vi "CheckKinect.vi"(8 "error in":errorcluster) -> (0 "error out":errorcluster, 2 "Hot?":bool)   [LabVIEW 2013]
doc: "Uses the Kinect to signal to the robot whether the goal is hot or not. If hands are detected, the goal is hot. Otherwise, the goal is not hot."
uses:
  <vilib>/addons/Kinect/Skeleton Vertex Index.ctl
  <vilib>/addons/Kinect/SkeletonVertexTrackState.ctl
panel:
  out "HandRightZ":sgl
  out "HandLeftZ":sgl
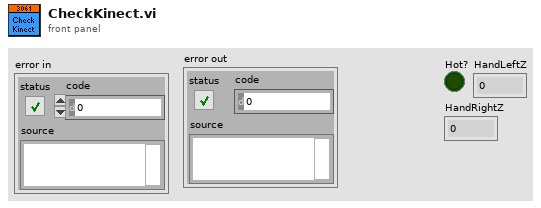
[diagram p1: front panel]
types:
  T1 = typedef "SkeletonVertexTrackState.ctl" = enum32{"NotTracked", "Inferred", "Tracked"}
  T2 = typedef "Skeleton Vertex Index.ctl" = i32
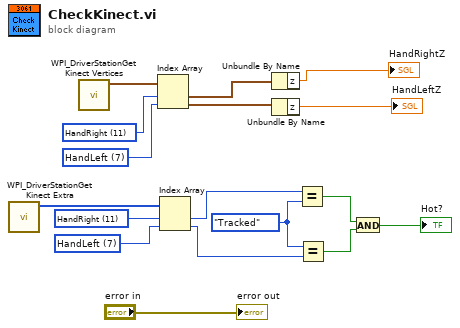
[diagram p0: block diagram]
diagram:
  w6 = SkeletonVertexTrackState."Tracked" ("x")
  w11 = T2 7 items=["HipCenter", "Spine", "ShoulderCenter", "Head", "ShoulderLeft", "ElbowLeft", "WristLeft", "HandLeft", "ShoulderRight", "ElbowRight", "WristRight", "HandRight", "HipLeft", "KneeLeft", "AnkleLeft", "FootLeft", "HipRight", "KneeRight", "AnkleRight", "FootRight"] ("Skeleton Joints")
  w12 = T2 11 items=["HipCenter", "Spine", "ShoulderCenter", "Head", "ShoulderLeft", "ElbowLeft", "WristLeft", "HandLeft", "ShoulderRight", "ElbowRight", "WristRight", "HandRight", "HipLeft", "KneeLeft", "AnkleLeft", "FootLeft", "HipRight", "KneeRight", "AnkleRight", "FootRight"] ("Skeleton Joints")
  w15 = T2 7 items=["HipCenter", "Spine", "ShoulderCenter", "Head", "ShoulderLeft", "ElbowLeft", "WristLeft", "HandLeft", "ShoulderRight", "ElbowRight", "WristRight", "HandRight", "HipLeft", "KneeLeft", "AnkleLeft", "FootLeft", "HipRight", "KneeRight", "AnkleRight", "FootRight"] ("Skeleton Joints")
  w16 = T2 11 items=["HipCenter", "Spine", "ShoulderCenter", "Head", "ShoulderLeft", "ElbowLeft", "WristLeft", "HandLeft", "ShoulderRight", "ElbowRight", "WristRight", "HandRight", "HipLeft", "KneeLeft", "AnkleLeft", "FootLeft", "HipRight", "KneeRight", "AnkleRight", "FootRight"] ("Skeleton Joints")
  n1 = call <vilib>:"WPI_DriverStationGet Kinect Extra.vi"() -> ("Skeleton Tracking State"=w17:T1[])  [unwired: 7 in, 4 out]
  n2 = call <vilib>:"WPI_DriverStationGet Kinect Vertices.vi"() -> ("Skeleton Vertices"=w13:cluster{"x":sgl, "y":sgl, "z":sgl}[])  [unwired: 10 in, 1 out]
  n3 = Index Array(array=w13, index #1=w12, index #2=w11) -> (element #1=w10:cluster{"x":sgl, "y":sgl, "z":sgl}, element #2=w9:cluster{"x":sgl, "y":sgl, "z":sgl})
  n4 = Index Array(array=w17, index #1=w16, index #2=w15) -> (element #1=w8:T1, element #2=w7:T1)
  n5 = Unbundle By Name(w10) -> ("z"=→"HandRightZ":sgl)
  n6 = Unbundle By Name(w9) -> ("z"=→"HandLeftZ":sgl)
  n7 = Equal?(x=w8, y=w6) -> (x = y?=w5:bool)
  n8 = Equal?(x=w6, y=w7) -> (x = y?=w4:bool)
  n9 = And(x=w5, y=w4) -> (x .and. y?=→"Hot?":bool)
  "error out" <- "error in"
